vi "Hub Centric Teleop Emulator.vi"(10 "Current Pose":cluster{"x":dbl, "y":dbl, "theta":dbl}, 11 "device ID":refnum<k1>) -> (3 "Robot Velocities":T1)   [LabVIEW 2020]
uses:
  <vilib>/Analysis/NI_AALPro.lvlib
  <vilib>/Analysis/_algsub.llb/Real Vector Norm.vi
  <vilib>/Analysis/coordinate.llb/2D Cartesian Coordinate Rotation (Scalar).vi
  swerve/Type Definitions/Data/Robot Velocities.ctl
panel:
  in  "Max Velocities":T2={"v(theta hub)"=10.0, "vr"=10.0, "v(theta robot)"=180.0}
  in  "Deadband":dbl=0.1
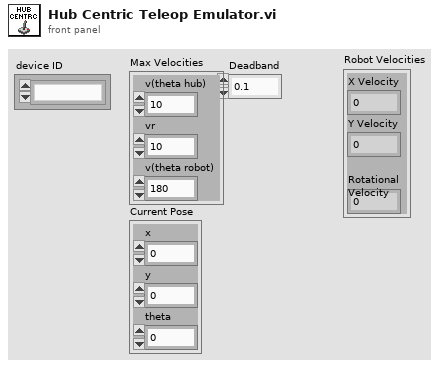
[diagram p1: front panel]
types:
  T1 = typedef "Robot Velocities.ctl" = cluster{"X Velocity":dbl, "Y Velocity":dbl, "Rotational \nVelocity":dbl}
  T2 = cluster{"v(theta hub)":dbl, "vr":dbl, "v(theta robot)":dbl}
  T3 = cluster{"X axis":i32, "Y axis":i32, "Z axis":i32, "X axis rotation":i32, "Y axis rotation":i32, "Z axis rotation":i32, "U axis":i32, "V axis":i32}
  T4 = cluster{"X axis":dbl, "Y axis":dbl, "Z axis":dbl, "X axis rotation":dbl, "Y axis rotation":dbl, "Z axis rotation":dbl, "U axis":dbl, "V axis":dbl}
  T5 = cluster{"X axis":dbl, dbl, "X axis rotation":dbl}
  T6 = cluster{"X axis":bool, bool, "X axis rotation":bool}
  T7 = cluster{"X axis":i16, i16, "X axis rotation":i16}
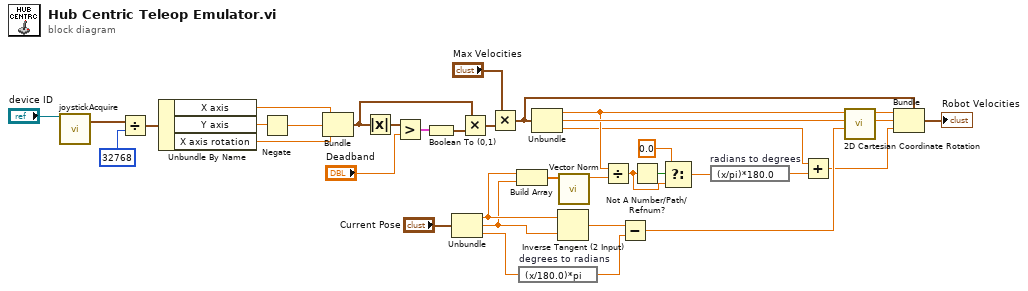
[diagram p0: block diagram]
diagram:
  n1 = call <vilib>:"joystickAcquire.vi"("device ID"="device ID") -> ("axis info"=w36:T3)  [unwired: 14 in, 4 out]
  n2 = Divide(x=w36, y=32768 ("X axis")) -> (x/y=w34:T4)
  n3 = Unbundle By Name(w34) -> ("X axis"=w32:dbl, "Y axis"=w30:dbl, "X axis rotation"=w31:dbl)
  n4 = Negate(x=w30) -> (-x=w29:dbl)
  n5 = Bundle("X axis"=w32, w29, "X axis rotation"=w31) -> (w24:T5)  [unwired: 1 in]
  n6 = Absolute Value(x=w24) -> (abs(x)=w28:T5)
  n7 = Greater?(x=w28, y="Deadband") -> (0:w26:T6)
  n8 = Boolean To (0,1)(Boolean=w26) -> (0, 1=w25:T7)
  n9 = Unbundle("Current Pose") -> ("x"=w13:dbl, "y"=w12:dbl, "theta"=w21:dbl)
  n10 = Multiply(x=w24, y=w25) -> (x*y=w23:T5)
  n11 = Multiply(x="Max Velocities", y=w23) -> (x*y=w16:cluster{dbl, dbl, dbl})
  n12 = Build Array(w13, w12) -> (w11:dbl[])
  n13 = expression code="(x/180.0)*pi" "degrees to radians"(w21) -> (w20:dbl)
  n14 = Unbundle(w16) -> (w7:dbl, w9:dbl, w1:dbl)
  n15 = Inverse Tangent (2 Input)(1:w12, 2:w13) -> (0:w14:dbl)
  n16 = call-poly <vilib>:"Vector Norm.vi"("Input Vector"=w11) -> ("norm"=w10:dbl)  [unwired: 9 in, 1 out]
  n17 = Divide(x=w7, y=w10) -> (x/y=w4:dbl)
  n18 = Subtract(x=w14, y=w20) -> (x-y=w19:dbl)
  n19 = Not A Number/Path/Refnum?(number/path/refnum=w4) -> (NaN/Path/Refnum?=w6:bool)
  n20 = Select(t=0.0, s=w6, f=w4) -> (s? t:f=w3:dbl)
  n21 = expression code="(x/pi)*180.0" "radians to degrees"(w3) -> (w2:dbl)
  n22 = Add(x=w1, y=w2) -> (x+y=w8:dbl)
  n23 = call-poly <vilib>:"2D Cartesian Coordinate Rotation.vi"("theta"=w19, "y"=w9, "x"=w7) -> ("y out"=w17:dbl, "x out"=w18:dbl)  [unwired: 6 in, 1 out]
  n24 = Bundle(cluster=w16, w18, w17, w8) -> (→"Robot Velocities":cluster{dbl, dbl, dbl})
